vi "Destroy.vi"(8 "error in (no error)":errorcluster, 11 "BME280 in":refnum<class "BME280.lvclass">) -> (0 "error out":errorcluster)   [LabVIEW 2020, in "BME280.lvclass"]
uses:
  BME280.lvclass
  BME280.lvclass/BME280.ctl
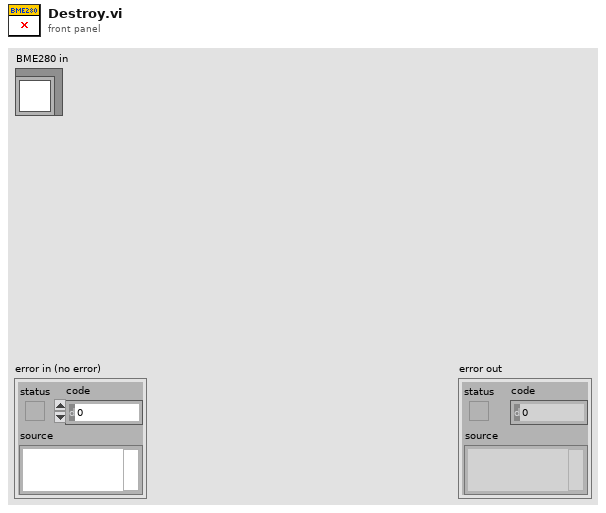
[diagram p1: front panel]
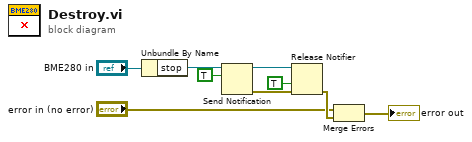
[diagram p0: block diagram]
diagram:
  n1 = Unbundle By Name("BME280 in") -> ("stop"=w8:refnum<notifier>)
  n2 = Send Notification(notification=TRUE, notifier=w8) -> (notifier out=w6:refnum<notifier>, error out=w5:errorcluster)  [unwired: 1 in]
  n3 = Release Notifier(notifier=w6, force destroy? (F)=TRUE, error in (no error)=w5) -> (error out=w3:errorcluster)  [unwired: 2 out]
  n4 = Merge Errors("error in (no error)", w3) -> (→"error out":errorcluster)
